vi "py.vi"() -> ()   [LabVIEW 2019]
panel:
  out "Numeric 2":dbl
  in  "Numeric":dbl
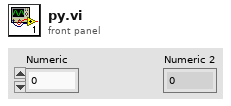
[diagram p1: front panel]
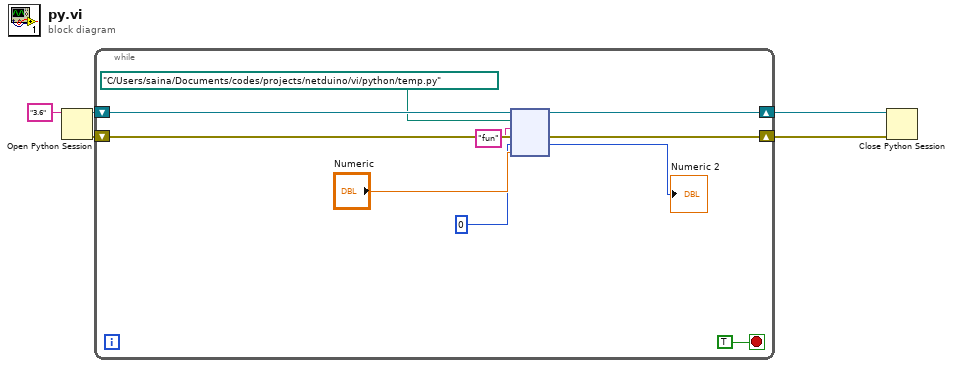
[diagram p0: block diagram]
diagram:
  n1 = Open Python Session(python version="3.6" ("Python version")) -> (session out=w4:refnum<k35>, error out=w3:errorcluster)  [unwired: 2 in]
  n2 = while {
    shift-right: [w10] -> w2
    shift-left: w4 -> [w15]
    shift-right: [w9] -> w1
    shift-left: w3 -> [w14]
    stop <- TRUE stop-if-true
    n3 = node(w15, path "C:/Users/saina/Documents/codes/projects/netduino/vi/python/temp.py" ("module path"), "fun" ("function name"), w14, 0, "Numeric") -> (w10:refnum<k35>, w9:errorcluster, →"Numeric 2":i32)  [unwired: 1 in, 2 out]
  }
  n4 = Close Python Session(session in=w2, error in=w1) -> ()  [unwired: 1 out]
